vi "Activity Light - Set Pulse Duration.vi"(8 "error in (no error)":errorcluster, 10 "Duration(ms)":u32=100, 11 "Name":string="Activity Light") -> (0 "error out":errorcluster)   [LabVIEW 2024, in "EQMF.lvlib" / "Status Utils.lvlib"]
uses:
  Status Utils.lvlib
  _Private/Activity Light Q Item.ctl
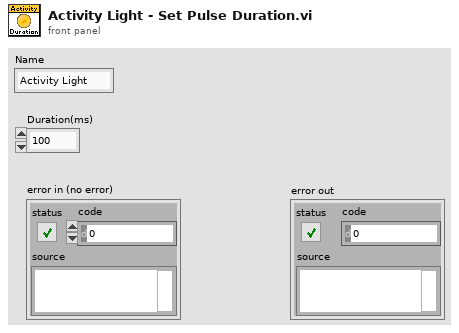
[diagram p1: front panel]
types:
  T1 = typedef "EQMF.lvlib/Status Utils.lvlib/Activity Light Q Item.ctl" = cluster{"Cmd":string, "Data":variant}
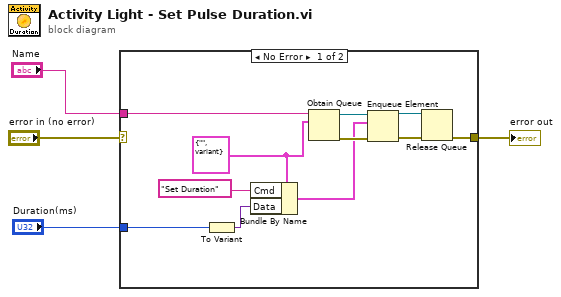
[diagram p0: block diagram]
diagram:
  n1 = case shown="No Error" "error in (no error)" {
    selector: "error in (no error)" -> [_ w16]
    tunnel: [w11 w16] -> w4
    tunnel: "Duration(ms)" -> [w6 _]
    tunnel: "Name" -> [w5 _]
    frame No Error {
      w9 = T1 {"Cmd"="", "Data"=variant} ("output cluster")
      n2 = To Variant(anything=w6) -> (Variant=w8:variant)
      n3 = Bundle By Name(cluster=w9, "Cmd"="Set Duration", "Data"=w8) -> (w7:T1)
      n4 = Obtain Queue(name (unnamed)=w5, element data type=w9) -> (queue out=w15:refnum<queue>, error out=w14:errorcluster)  [unwired: 3 in, 1 out]
      n5 = Enqueue Element(queue=w15, element=w7, error in (no error)=w14) -> (queue out=w12:refnum<queue>, error out=w13:errorcluster)  [unwired: 1 in, 1 out]
      n6 = Release Queue(queue=w12, error in (no error)=w13) -> (error out=w11:errorcluster)  [unwired: 1 in, 2 out]
    }
    frame Error {
    }
  }
  "error out" <- w4
